vi "PWM_SetValue.vi"(0 "FPGA_Ref_in":refnum<k20>, 5 "PWM":T1=1 items=["Invalid"=0, "PWM1"=1, "PWM2"=2, "PWM9"=9, "PWM10"=10], 7 "High (uSec)":u32, 9 "Period (uSec)":u32, 11 "error in":errorcluster) -> (4 "FPGA_Ref_out":refnum<k20>, 15 "error out":errorcluster)   [LabVIEW 2009, in "PWM.lvlib"]
uses:
  PWM.lvlib
  PWM_Name.ctl
  <vilib>/rvi/interface/nirviReadWriteControl/nirviReadWriteControl.xnode
  FPGA Bitfiles/scmproject.lvproj_FPGA Target_RobotFPGA.vi.lvbitx
  RobotFPGA.vi
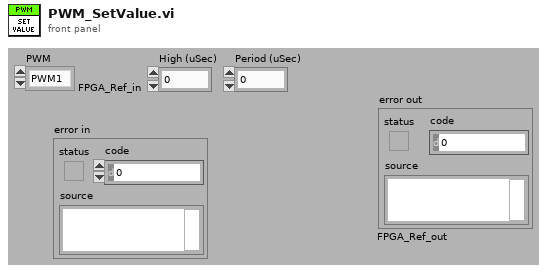
[diagram p1: front panel]
types:
  T1 = typedef "PWM.lvlib/PWM_Name.ctl" = u16
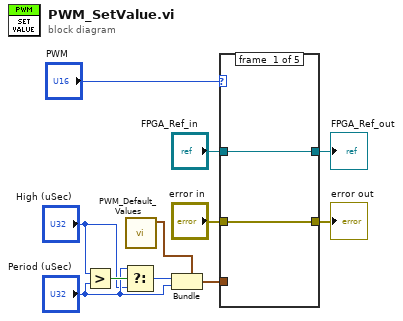
[diagram p0: block diagram]
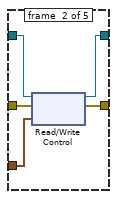
[diagram p2: hidden frame]
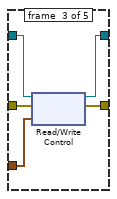
[diagram p3: hidden frame]
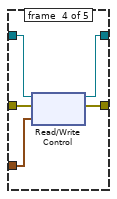
[diagram p4: hidden frame]
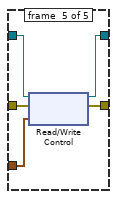
[diagram p5: hidden frame]
diagram:
  n1 = Greater?(x="High (uSec)", y="Period (uSec)") -> (0:w5:bool)
  n2 = Select(t="Period (uSec)", s=w5, f="High (uSec)") -> (s? t:f=w6:u32)
  n3 = call "PWM_Default_Values.vi"() -> ("PWM_default"=w7:cluster{"High (uSec)":u32, "Period (uSec)":u32})  [unwired: 11 in]
  n4 = Bundle(cluster=w7, "High (uSec)"=w6, "Period (uSec)"="Period (uSec)") -> (w8:cluster{"High (uSec)":u32, "Period (uSec)":u32})
  n5 = case shown="1" "PWM" {
    tunnel: "FPGA_Ref_in" -> [w13 w15 w33 w51 w69]
    tunnel: "error in" -> [w12 w18 w36 w54 w72]
    tunnel: [w13 w14 w32 w50 w68] -> w2
    tunnel: [w12 w17 w35 w53 w71] -> w1
    tunnel: w8 -> [_ w16 w34 w52 w70]
    frame #0 {
    }
    frame #1 {
      n6 = xnode "Read/Write Control"("FPGA VI Reference In"=w15, "error in"=w18, "PWM1"=w16) -> ("FPGA VI Reference Out"=w14:refnum<k20>, "error out"=w17:errorcluster)
    }
    frame #2 {
      n7 = xnode "Read/Write Control"("FPGA VI Reference In"=w33, "error in"=w36, "PWM2"=w34) -> ("FPGA VI Reference Out"=w32:refnum<k20>, "error out"=w35:errorcluster)
    }
    frame #3 {
      n8 = xnode "Read/Write Control"("FPGA VI Reference In"=w51, "error in"=w54, "PWM9"=w52) -> ("FPGA VI Reference Out"=w50:refnum<k20>, "error out"=w53:errorcluster)
    }
    frame #4 {
      n9 = xnode "Read/Write Control"("FPGA VI Reference In"=w69, "error in"=w72, "PWM10"=w70) -> ("FPGA VI Reference Out"=w68:refnum<k20>, "error out"=w71:errorcluster)
    }
  }
  "error out" <- w1
  "FPGA_Ref_out" <- w2
